vi "Gen_Random_Sine.vi"() -> (3 "data":dbl[](graph))   [LabVIEW 2020]
uses:
  <vilib>/measure/NI_MABase.lvlib
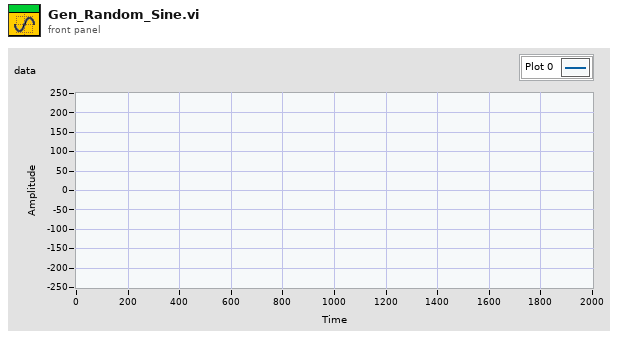
[diagram p1: front panel]
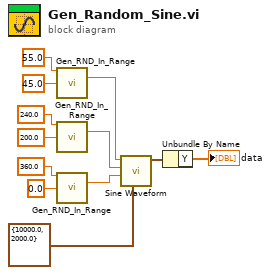
[diagram p0: block diagram]
diagram:
  n1 = call "Gen_RND_In_Range.vi"("Upper Bound"=55.0 ("frequency"), "Lower Bound"=45.0 ("Variation%")) -> ("RND_In_Range"=w9:dbl)  [unwired: 13 in]
  n2 = call "Gen_RND_In_Range.vi"("Upper Bound"=240.0 ("amplitude"), "Lower Bound"=200.0 ("variation")) -> ("RND_In_Range"=w7:dbl)  [unwired: 13 in]
  n3 = call "Gen_RND_In_Range.vi"("Upper Bound"=360.0 ("phase(digree)"), "Lower Bound"=0.0 ("Range")) -> ("RND_In_Range"=w12:dbl)  [unwired: 13 in]
  n4 = call <vilib>:"Sine Waveform.vi"("sampling info"=cluster{"Fs":dbl, "#s":dbl} {"Fs"=10000.0, "#s"=2000.0} ("sampling info for sine"), "phase"=w12, "amplitude"=w7, "frequency"=w9) -> ("signal out"=w11:waveform(dbl))  [unwired: 6 in, 1 out]
  n5 = Unbundle By Name(w11) -> ("Y"=→"data":dbl[])
